vi "interactive control.vi"() -> ()   [LabVIEW 2010]
panel:
  in  "Write Data":string
  out "Read Data":string
  in  "GPIB Address":string
  # "COMMANDS CASE DEPENDENT\nH-Heater\nI:Setpoint\nA:Activity(0hold,1toset,2tozero,4clamp)\nS:Setrate\nR0:leads current\nR1:PS voltage\nR16:persistent current"
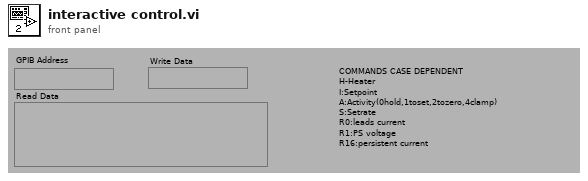
[diagram p1: front panel]
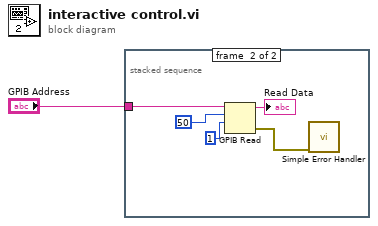
[diagram p0: block diagram]
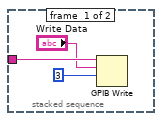
[diagram p2: hidden frame]
diagram:
  n1 = stacked-sequence {
    tunnel: "GPIB Address" -> [w4 w9]
    frame #0 {
      n2 = GPIB Write(0:w4, 1:"Write Data", 2:i16 3 ("mode (0)")) -> ()  [unwired: 2 in, 2 out]
    }
    frame #1 {
      n3 = GPIB Read(0:w9, 1:50 ("byte count"), 2:i16 1 ("mode (0)")) -> (5:→"Read Data":string, 7:w6:errorcluster)  [unwired: 2 in, 1 out]
      n4 = call <vilib>:"Simple Error Handler.vi"("error in (no error)"=w6) -> ()  [unwired: 4 in, 5 out]
    }
  }
